vi "Opgave 3 Stoerste tal.vi"(11 "Antal tal":i32) -> (2 "Alle tal":dbl[](array[numeric]), 3 "Max værdi":dbl)   [LabVIEW 2019]
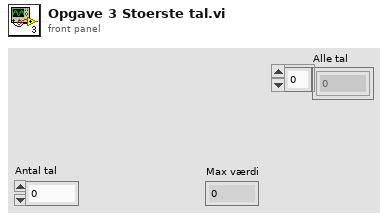
[diagram p1: front panel]
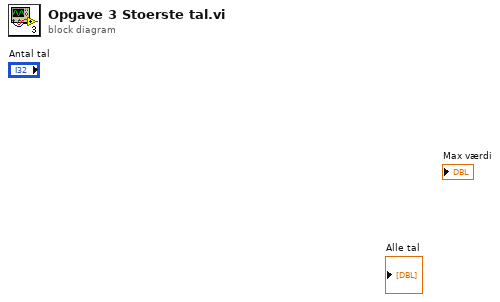
[diagram p0: block diagram]
diagram:
